vi "zad_5_b.vi"() -> ()   [LabVIEW 2025]
uses:
  <vilib>/numeric/Random Number (Range) I64.vi
  <vilib>/numeric/sub_Random U32.vi
panel:
  out "error out":errorcluster
  in  "error in":errorcluster
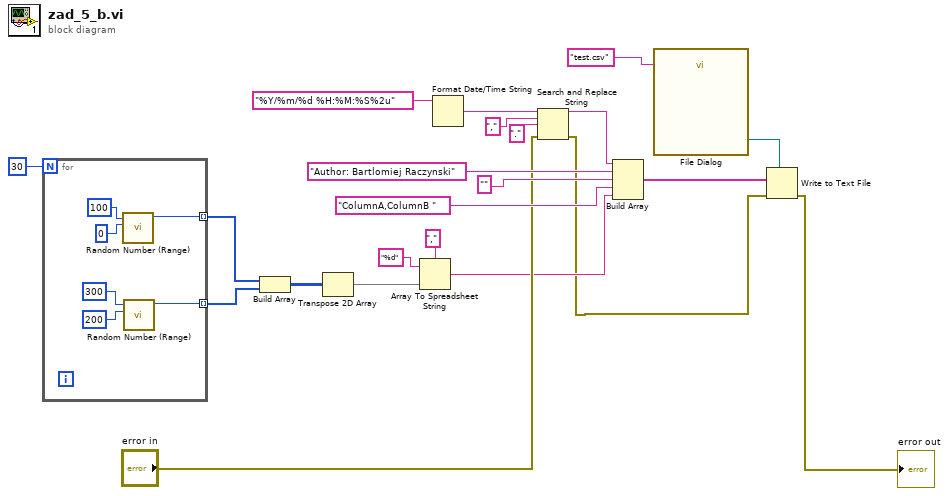
[diagram p0: block diagram]
diagram:
  n1 = for {
    N: 30 -> [_]
    tunnel: [w23] -> w17 mode=indexing
    tunnel: [w24] -> w18 mode=indexing
    n2 = call-poly <vilib>:"Random Number (Range).vi"("lower bound (-100)"=i64 0 ("lower bound (0)"), "upper bound (100)"=i64 100) -> ("number"=w23:i64)  [unwired: 9 in]
    n3 = call-poly <vilib>:"Random Number (Range).vi"("lower bound (-100)"=i64 200 ("lower bound (0)"), "upper bound (100)"=i64 300) -> ("number"=w24:i64)  [unwired: 9 in]
  }
  n4 = Build Array(w17, w18) -> (w6:i64[][])
  n5 = Transpose 2D Array(2D array=w6) -> (transposed array=w4:i64[][])
  n6 = Array To Spreadsheet String(delimiter (Tab)=",", array=w4, 3:"%d" ("format string")) -> (spreadsheet string=w5:string)
  n7 = Format Date/Time String(time format string (%c)="%Y/%m/%d %H:%M:%S%2u") -> (date/time string=w13:string)  [unwired: 2 in]
  n8 = Search and Replace String(input string=w13, search string=",", replace string="." ("replace string (\"\")"), error in="error in") -> (result string=w10:string, error out=w3:errorcluster)  [unwired: 4 in, 2 out]
  n9 = Build Array(w10, "Author: Bartlomiej Raczynski", "" ("element"), "ColumnA,ColumnB ", w5) -> (w12:string[])
  n10 = call "File Dialog"("default name"="test.csv") -> ("selected path"=w11:path)  [unwired: 11 in, 3 out]
  n11 = Write to Text File(file (use dialog)=w11, text=w12, error in=w3) -> (error out=→"error out":errorcluster)  [unwired: 1 in, 2 out]
